vi "Boonton7200_Write_GPIB.vi"(7 "GPIB Address String":string="18", 8 "Error In":errorcluster, 9 "Special Functions":T1, 10 "Data Value":sgl, 11 "IEEE-488 Bus Mnemonics":T2) -> (0 "Error Out":errorcluster)   [LabVIEW 2015, in "Boonton7200.lvlib"]
uses:
  Boonton7200.lvlib
  Boonton7200_IEEE-488_Bus_Mnemonics.ctl
  Boonton7200_Special_Function_Codes.ctl
panel:
  out "GPIB code (IEEE-488)":string
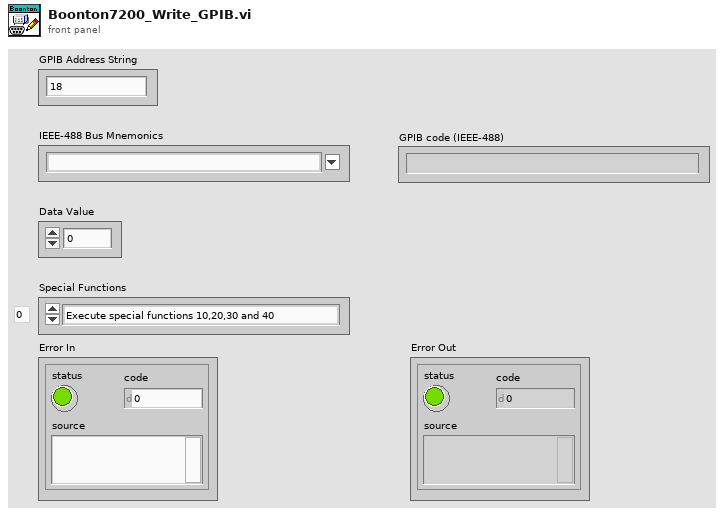
[diagram p1: front panel]
types:
  T1 = typedef "Boonton7200_Special_Function_Codes.ctl" = enum16{"Execute special functions 10,20,30 and 40", "Test Level display and entry", "Capacitance Standard display and entry", "Conductance Standard dispaly and entry", "Capacitance Low Limit display and entry", "Capacitance High Limit dispaly and entry", "IEEE-488 Bus Address display and entry", "End-of-string charecter display and selection", "Capacitance uncertainty display", "Conductance uncertainty dispaly", "Automatic selection(Measurement Ranging Functions)", "Hold current measurement range", "Set and hold 2.000 pF / 2.00 uS range", "Set and hold 20.00 pF / 20.0 uS range", "Set and hold 200.0 pF / 200 uS range", "Set and holde 2000 pF / 2000 uS range", "16 - Not Defined", "17 - Not Defined", "18 - Not Defined", "19 - Not Defined", "Automatic selection(Internal Bias Ranging Functions)", "Hold current bias range", "Set and hold 20.000 V range", "Set and Hold 100.00 V range", "24 - Not Defined", "25 - Not Defined", "26 - Not Defined", "27 - Not Defined", "28 - Not Defined", "29 - Not Defined", "30 Automatic selection(Measurement Filter Functions)", "Filter length = 1 measurement, no average", "Filter length = 2 measurement", "Filter length = 5 measurement", "Filter length = 10 measurement", "Filter length = 20 measurement", "Filter length = 50 measurement", "Filter length = 100 measurement", "Filter length = 200 measurement", "Filter length = 500 measurement", "Normal operation, free-run dispaly(Sercvice Request Functions)", "Disable SRQ interrupt", "Enable SRQ interrupt", "Set SRQ mask when an error occurs", "Set SRQ mask and update dispaly when measurement filter is complete", "Set SRQ mask when capacitance measurement is within the high and low limit settings", "Set SRQ mask when capacitance measurement exceeds the high or low limit settings", "Set SRQ mask when zero or calibration is complete", "Set SRQ mask when sweep is complete", "49 - Not Defined", "Calibrate detector offset(Automatic Calibration and Test Functions)", "Calibrate external bias offset", "Calibrate internal bias offset", "Calibrate full-scale capacitance", "Calibrate conductance phase", "Display internal temperature", "Display amplitude error due to temperature influence", "Display phase error due to temperature influence", "Initialize instrument and erase all program locations", "Initalize software calibration variables"}
  T2 = typedef "Boonton7200_IEEE-488_Bus_Mnemonics.ctl" = string
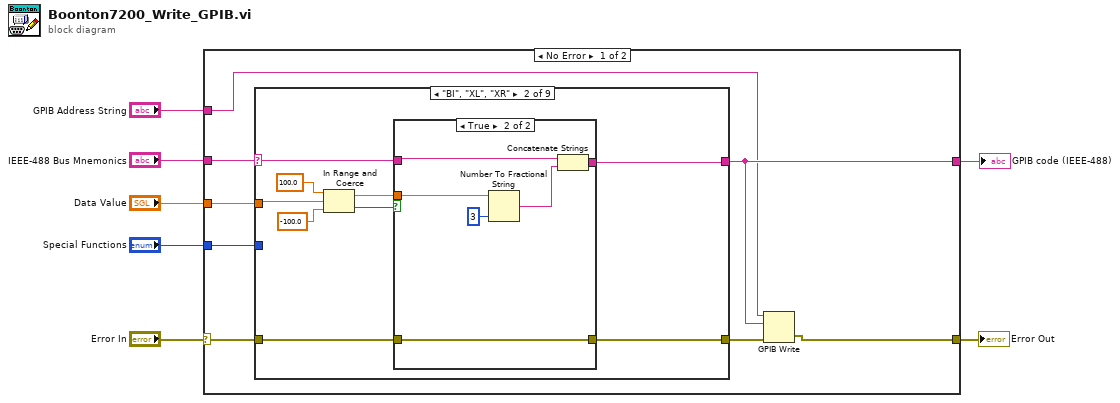
[diagram p0: block diagram]
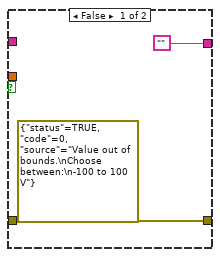
[diagram p3: hidden frame]
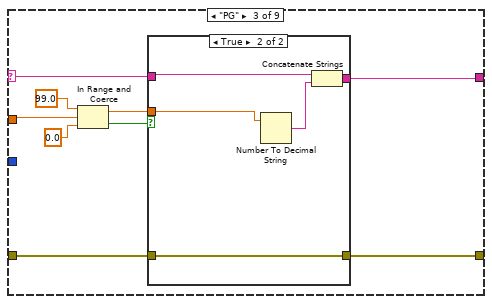
[diagram p4: hidden frame]
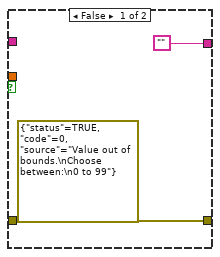
[diagram p5: hidden frame]
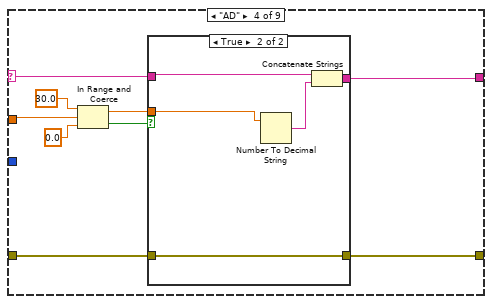
[diagram p6: hidden frame]
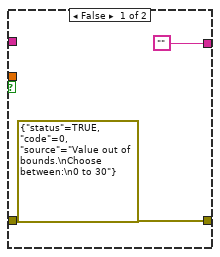
[diagram p7: hidden frame]
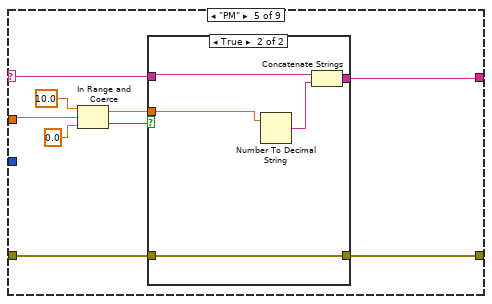
[diagram p8: hidden frame]
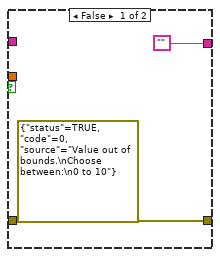
[diagram p9: hidden frame]
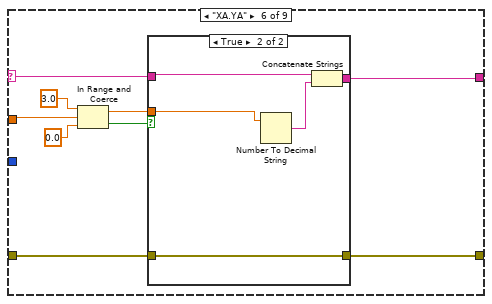
[diagram p10: hidden frame]
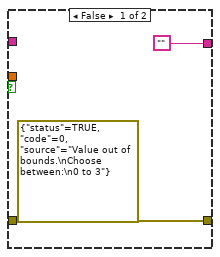
[diagram p11: hidden frame]
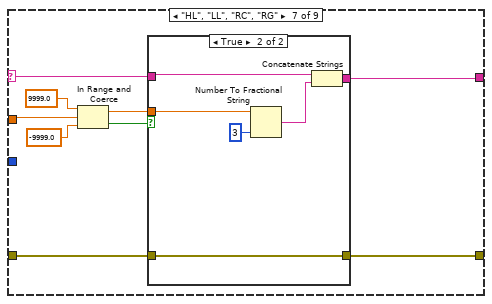
[diagram p12: hidden frame]
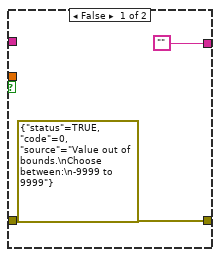
[diagram p13: hidden frame]
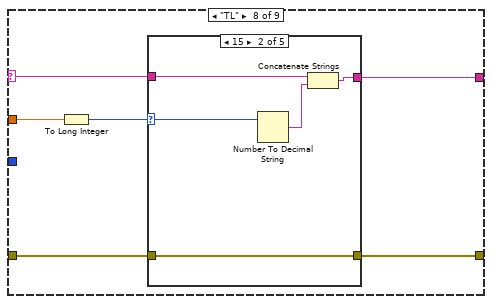
[diagram p14: hidden frame]
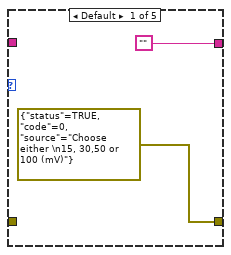
[diagram p15: hidden frame]
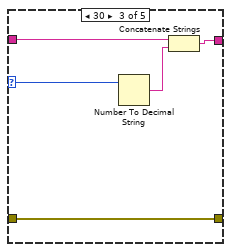
[diagram p16: hidden frame]
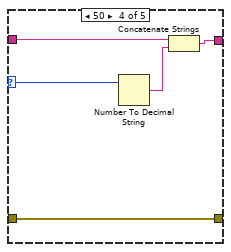
[diagram p17: hidden frame]
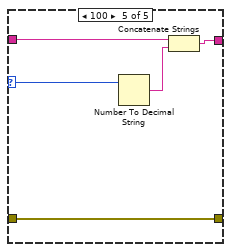
[diagram p18: hidden frame]
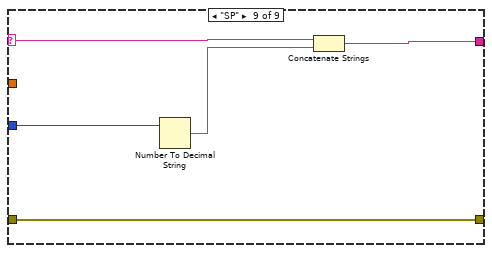
[diagram p19: hidden frame]
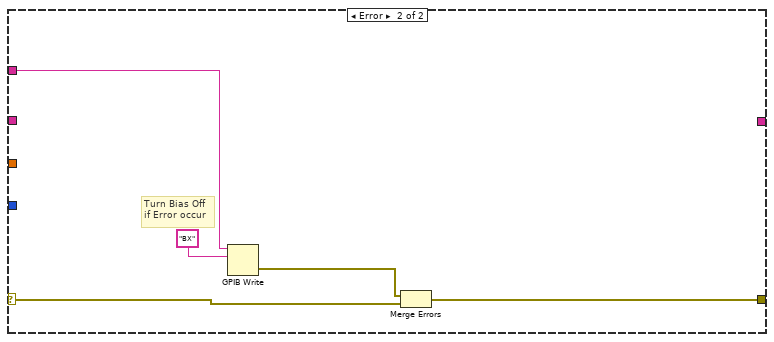
[diagram p20: hidden frame]
diagram:
  n1 = case shown="No Error" "Error In" {
    selector: "Error In" -> [w14 w149]
    tunnel: [w8 w151] -> w6
    tunnel: "IEEE-488 Bus Mnemonics" -> [w15 _]
    tunnel: [w11 _] -> w4
    tunnel: "Data Value" -> [w13 _]
    tunnel: "Special Functions" -> [w12 _]
    tunnel: "GPIB Address String" -> [w9 w153]
    frame No Error {
      n2 = case shown="\"BI\", \"XL\", \"XR\"" w15 {
        selector: w15 -> [w16 w19 w36 w52 w68 w84 w100 w119 w147]
        tunnel: w14 -> [w17 w26 w43 w59 w75 w91 w107 w121 w144]
        tunnel: [w17 w25 w42 w58 w74 w90 w106 w120 w144] -> w10
        tunnel: [w16 w18 w35 w51 w67 w83 w99 w118 w148] -> w11
        tunnel: w13 -> [_ w24 w41 w57 w73 w89 w105 w116 _]
        tunnel: w12 -> [_ _ _ _ _ _ _ _ w145]
        frame Default {
        }
        frame "BI", "XL", "XR" {
          n3 = In Range and Coerce(upper limit=sgl 100.0, x=w24, lower limit=sgl -100.0) -> (coerced(x)=w20:sgl, In Range?=w21:bool)
          n4 = case shown="True" w21 {
            tunnel: w26 -> [_ w34]
            tunnel: [errorcluster {"status"=TRUE, "code"=0, "source"="Value out of bounds.\nChoose between:\n-100 to 100 V"} ("error constant") w34] -> w25
            tunnel: w20 -> [_ w30]
            tunnel: w19 -> [_ w31]
            tunnel: ["" w32] -> w18
            frame False {
            }
            frame True {
              n5 = Number To Fractional String(number=w30, precision (6)=i16 3) -> (F-format string=w33:string)  [unwired: 2 in]
              n6 = Concatenate Strings(w31, w33) -> (w32:string)
            }
          }
        }
        frame "PG" {
          n7 = In Range and Coerce(upper limit=sgl 99.0, x=w41, lower limit=sgl 0.0) -> (coerced(x)=w37:sgl, In Range?=w38:bool)
          n8 = case shown="True" w38 {
            tunnel: w43 -> [_ w50]
            tunnel: [errorcluster {"status"=TRUE, "code"=0, "source"="Value out of bounds.\nChoose between:\n0 to 99"} ("error constant") w50] -> w42
            tunnel: w37 -> [_ w46]
            tunnel: w36 -> [_ w47]
            tunnel: ["" w48] -> w35
            frame False {
            }
            frame True {
              n9 = Number To Decimal String(number=w46) -> (decimal integer string=w49:string)  [unwired: 1 in]
              n10 = Concatenate Strings(w47, w49) -> (w48:string)
            }
          }
        }
        frame "AD" {
          n11 = In Range and Coerce(upper limit=sgl 30.0, x=w57, lower limit=sgl 0.0) -> (coerced(x)=w53:sgl, In Range?=w54:bool)
          n12 = case shown="True" w54 {
            tunnel: w59 -> [_ w66]
            tunnel: [errorcluster {"status"=TRUE, "code"=0, "source"="Value out of bounds.\nChoose between:\n0 to 30"} ("error constant") w66] -> w58
            tunnel: w53 -> [_ w62]
            tunnel: w52 -> [_ w63]
            tunnel: ["" w64] -> w51
            frame False {
            }
            frame True {
              n13 = Number To Decimal String(number=w62) -> (decimal integer string=w65:string)  [unwired: 1 in]
              n14 = Concatenate Strings(w63, w65) -> (w64:string)
            }
          }
        }
        frame "PM" {
          n15 = In Range and Coerce(upper limit=sgl 10.0, x=w73, lower limit=sgl 0.0) -> (coerced(x)=w69:sgl, In Range?=w70:bool)
          n16 = case shown="True" w70 {
            tunnel: w75 -> [_ w82]
            tunnel: [errorcluster {"status"=TRUE, "code"=0, "source"="Value out of bounds.\nChoose between:\n0 to 10"} ("error constant") w82] -> w74
            tunnel: w69 -> [_ w78]
            tunnel: w68 -> [_ w79]
            tunnel: ["" w80] -> w67
            frame False {
            }
            frame True {
              n17 = Number To Decimal String(number=w78) -> (decimal integer string=w81:string)  [unwired: 1 in]
              n18 = Concatenate Strings(w79, w81) -> (w80:string)
            }
          }
        }
        frame "XA.YA" {
          n19 = In Range and Coerce(upper limit=sgl 3.0, x=w89, lower limit=sgl 0.0) -> (coerced(x)=w85:sgl, In Range?=w86:bool)
          n20 = case shown="True" w86 {
            tunnel: w91 -> [_ w98]
            tunnel: [errorcluster {"status"=TRUE, "code"=0, "source"="Value out of bounds.\nChoose between:\n0 to 3"} ("error constant") w98] -> w90
            tunnel: w85 -> [_ w94]
            tunnel: w84 -> [_ w95]
            tunnel: ["" w96] -> w83
            frame False {
            }
            frame True {
              n21 = Number To Decimal String(number=w94) -> (decimal integer string=w97:string)  [unwired: 1 in]
              n22 = Concatenate Strings(w95, w97) -> (w96:string)
            }
          }
        }
        frame "HL", "LL", "RC", "RG" {
          n23 = In Range and Coerce(upper limit=sgl 9999.0, x=w105, lower limit=sgl -9999.0) -> (coerced(x)=w101:sgl, In Range?=w102:bool)
          n24 = case shown="True" w102 {
            tunnel: w107 -> [_ w115]
            tunnel: [errorcluster {"status"=TRUE, "code"=0, "source"="Value out of bounds.\nChoose between:\n-9999 to 9999"} ("error constant") w115] -> w106
            tunnel: w101 -> [_ w110]
            tunnel: w100 -> [_ w113]
            tunnel: ["" w114] -> w99
            frame False {
            }
            frame True {
              n25 = Number To Fractional String(number=w110, precision (6)=i16 3) -> (F-format string=w111:string)  [unwired: 2 in]
              n26 = Concatenate Strings(w113, w111) -> (w114:string)
            }
          }
        }
        frame "TL" {
          n27 = To Long Integer(number=w116) -> (32bit integer=w117:i32)
          n28 = case shown="15" w117 {
            selector: w117 -> [_ w124 w129 w134 w139]
            tunnel: w121 -> [_ w128 w133 w138 w143]
            tunnel: [errorcluster {"status"=TRUE, "code"=0, "source"="Choose either \n15, 30,50 or 100 (mV)"} ("error constant") w128 w133 w138 w143] -> w120
            tunnel: w119 -> [_ w126 w131 w136 w141]
            tunnel: ["" w127 w132 w137 w142] -> w118
            frame Default {
            }
            frame 15 {
              n29 = Number To Decimal String(number=w124) -> (decimal integer string=w125:string)  [unwired: 1 in]
              n30 = Concatenate Strings(w126, w125) -> (w127:string)
            }
            frame 30 {
              n31 = Number To Decimal String(number=w129) -> (decimal integer string=w130:string)  [unwired: 1 in]
              n32 = Concatenate Strings(w131, w130) -> (w132:string)
            }
            frame 50 {
              n33 = Number To Decimal String(number=w134) -> (decimal integer string=w135:string)  [unwired: 1 in]
              n34 = Concatenate Strings(w136, w135) -> (w137:string)
            }
            frame 100 {
              n35 = Number To Decimal String(number=w139) -> (decimal integer string=w140:string)  [unwired: 1 in]
              n36 = Concatenate Strings(w141, w140) -> (w142:string)
            }
          }
        }
        frame "SP" {
          n37 = Number To Decimal String(number=w145) -> (decimal integer string=w146:string)  [unwired: 1 in]
          n38 = Concatenate Strings(w147, w146) -> (w148:string)
        }
      }
      n39 = GPIB Write(0:w9, 1:w11, 3:w10) -> (6:w8:errorcluster)  [unwired: 2 in, 1 out]
    }
    frame Error {
      # "Turn Bias Off\nif Error occur"
      n40 = GPIB Write(0:w153, 1:"BX" ("data")) -> (6:w150:errorcluster)  [unwired: 3 in, 1 out]
      n41 = Merge Errors(w150, w149) -> (w151:errorcluster)
    }
  }
  "Error Out" <- w6
  "GPIB code (IEEE-488)" <- w4
